vi "Add Authentication.vi"(7 "WSDL URL":string, 8 "error in (no error)":errorcluster, 9 "Proxy Server Settings":T1, 10 "Web Service Authentication":T2, 11 "SoapHttpClientProtocolIn":refnum<k24>) -> (0 "error out":errorcluster, 3 "SoapHttpClientProtocolOut":refnum<k24>)   [LabVIEW 2017, in "WebServiceImporter.lvlib" / "VI Generator.lvlib"]
uses:
  <vilib>/Platform/WebService/VI Generator/VI Generator.lvlib
  System.Web.Services
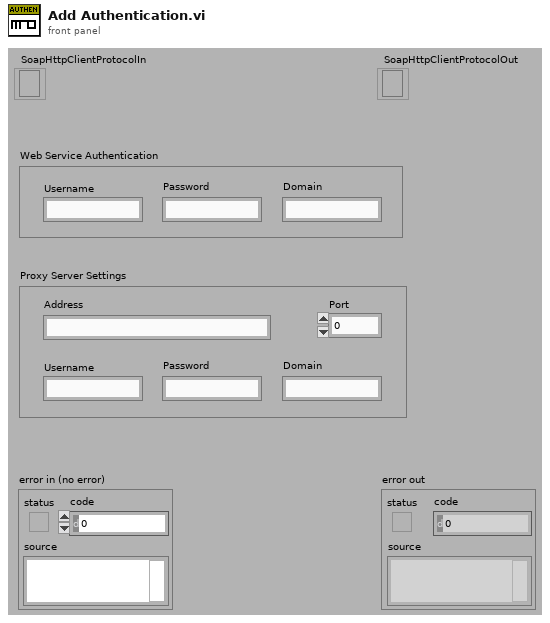
[diagram p1: front panel]
types:
  T1 = cluster{"Address":string, "Port":u32, "Username":string, "Password":string, "Domain":string}
  T2 = cluster{"Username":string, "Password":string, "Domain":string}
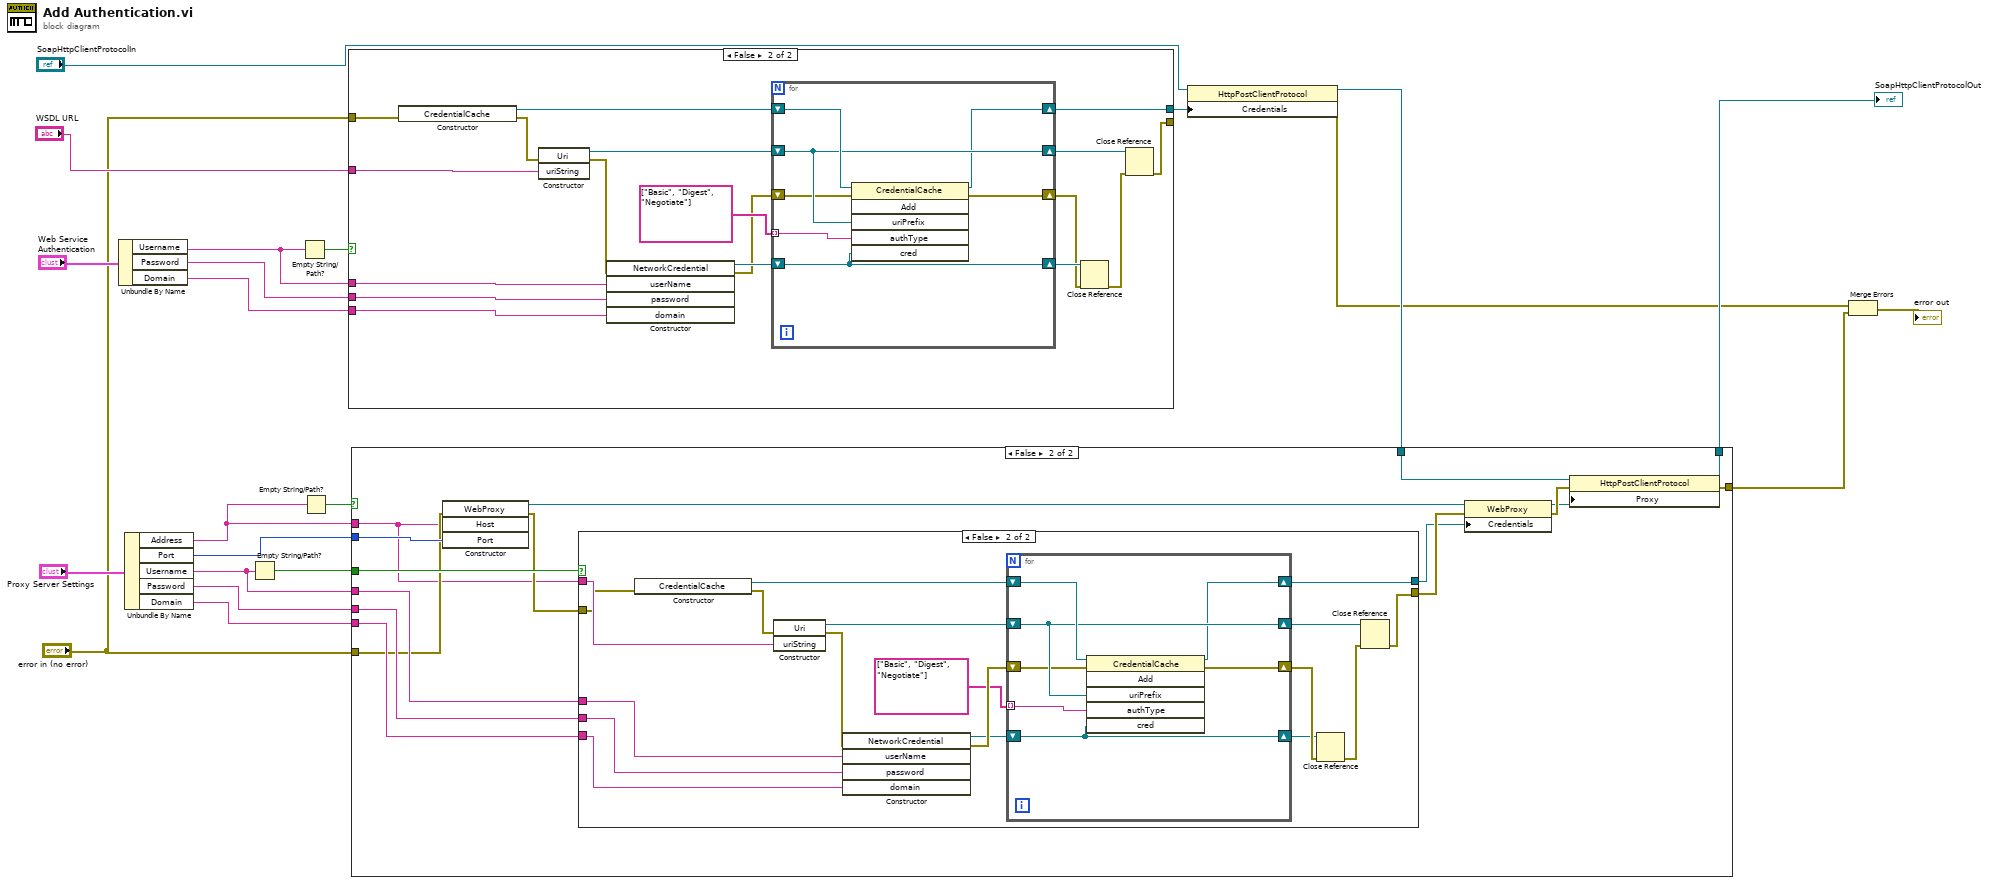
[diagram p0: block diagram]
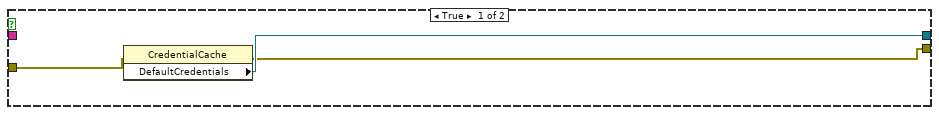
[diagram p3: hidden frame]
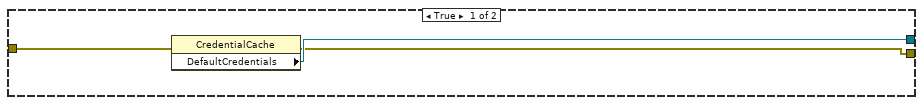
[diagram p4: hidden frame]
diagram:
  n1 = Unbundle By Name("Web Service Authentication") -> ("Username"=w18:string, "Password"=w17:string, "Domain"=w16:string)
  n2 = Unbundle By Name("Proxy Server Settings") -> ("Address"=w12:string, "Port"=w11:u32, "Username"=w7:string, "Password"=w9:string, "Domain"=w8:string)
  n3 = Empty String/Path?(string/path=w7) -> (empty?=w10:bool)
  n4 = Empty String/Path?(string/path=w18) -> (empty?=w20:bool)
  n5 = Empty String/Path?(string/path=w12) -> (empty?=w13:bool)
  n6 = case shown="False" w20 {
    tunnel: "error in (no error)" -> [w25 w43]
    tunnel: "WSDL URL" -> [_ w41]
    tunnel: w18 -> [_ w40]
    tunnel: w17 -> [_ w39]
    tunnel: w16 -> [_ w38]
    tunnel: [w23 w27] -> _
    tunnel: [w24 w26] -> w14
    frame True {
      n7 = property class="CredentialCache"(error in=w25) -> (error out=w23:errorcluster, "DefaultCredentials"=w24:refnum<k24>)  [unwired: 1 in, 1 out]
    }
    frame False {
      n8 = constructor class="CredentialCache"(error in=w43) -> (reference out=w35:refnum<k24>, error out=w42:errorcluster)  [unwired: 2 in, 1 out]
      n9 = constructor class="Uri"(error in=w42, "uriString"=w41) -> (reference out=w34:refnum<k24>, error out=w37:errorcluster)  [unwired: 2 in, 2 out]
      n10 = constructor class="NetworkCredential"(error in=w37, "userName"=w40, "password"=w39, "domain"=w38) -> (reference out=w33:refnum<k24>, error out=w32:errorcluster)  [unwired: 2 in, 4 out]
      n11 = for {
        tunnel: string[] ["Basic", "Digest", "Negotiate"] -> [w45] mode=indexing
        shift-right: [w46] -> w28
        shift-left: w32 -> [w47]
        shift-right: [w49] -> w30
        shift-left: w34 -> [w49]
        shift-right: [w48] -> w26
        shift-left: w35 -> [w50]
        shift-right: [w44] -> w31
        shift-left: w33 -> [w44]
        n12 = invoke class="CredentialCache" method="Add"(reference=w50, error in=w47, "uriPrefix"=w49, "authType"=w45, "cred"=w44) -> (reference out=w48:refnum<k24>, error out=w46:errorcluster)  [unwired: 1 in, 4 out]
      }
      n13 = Close Reference(reference=w31, error in (no error)=w28) -> (error out=w29:errorcluster)
      n14 = Close Reference(reference=w30, error in (no error)=w29) -> (error out=w27:errorcluster)
    }
  }
  n15 = property class="HttpPostClientProtocol"(reference="SoapHttpClientProtocolIn", "Credentials"=w14) -> (reference out=w5:refnum<k24>, error out=w3:errorcluster)  [unwired: 1 in]
  n16 = case shown="False" w13 {
    tunnel: w12 -> [_ w61]
    tunnel: w11 -> [_ w68]
    tunnel: w10 -> [_ w67]
    tunnel: w9 -> [_ w65]
    tunnel: w8 -> [_ w64]
    tunnel: w7 -> [_ w66]
    tunnel: "error in (no error)" -> [w51 w63]
    tunnel: w5 -> [w52 w57]
    tunnel: [w52 w55] -> w4
    tunnel: [w51 w54] -> w2
    frame True {
    }
    frame False {
      n17 = constructor class="WebProxy"(error in=w63, "Host"=w61, "Port"=w68) -> (reference out=w58:refnum<k24>, error out=w62:errorcluster)  [unwired: 2 in, 3 out]
      n18 = case shown="False" w67 {
        tunnel: w66 -> [_ w76]
        tunnel: w65 -> [_ w75]
        tunnel: w64 -> [_ w74]
        tunnel: w62 -> [w71 w77]
        tunnel: w61 -> [_ w78]
        tunnel: [w69 w73] -> w60
        tunnel: [w70 w72] -> w59
        frame True {
          n19 = property class="CredentialCache"(error in=w71) -> (error out=w69:errorcluster, "DefaultCredentials"=w70:refnum<k24>)  [unwired: 1 in, 1 out]
        }
        frame False {
          n20 = constructor class="CredentialCache"(error in=w77) -> (reference out=w82:refnum<k24>, error out=w79:errorcluster)  [unwired: 2 in, 1 out]
          n21 = constructor class="Uri"(error in=w79, "uriString"=w78) -> (reference out=w83:refnum<k24>, error out=w80:errorcluster)  [unwired: 2 in, 2 out]
          n22 = constructor class="NetworkCredential"(error in=w80, "userName"=w76, "password"=w75, "domain"=w74) -> (reference out=w84:refnum<k24>, error out=w85:errorcluster)  [unwired: 2 in, 4 out]
          n23 = for {
            tunnel: string[] ["Basic", "Digest", "Negotiate"] -> [w91] mode=indexing
            shift-right: [w92] -> w89
            shift-left: w85 -> [w93]
            shift-right: [w95] -> w87
            shift-left: w83 -> [w95]
            shift-right: [w94] -> w72
            shift-left: w82 -> [w96]
            shift-right: [w90] -> w86
            shift-left: w84 -> [w90]
            n24 = invoke class="CredentialCache" method="Add"(reference=w96, error in=w93, "uriPrefix"=w95, "authType"=w91, "cred"=w90) -> (reference out=w94:refnum<k24>, error out=w92:errorcluster)  [unwired: 1 in, 4 out]
          }
          n25 = Close Reference(reference=w86, error in (no error)=w89) -> (error out=w88:errorcluster)
          n26 = Close Reference(reference=w87, error in (no error)=w88) -> (error out=w73:errorcluster)
        }
      }
      n27 = property class="WebProxy"(reference=w58, error in=w60, "Credentials"=w59) -> (reference out=w53:refnum<k24>, error out=w56:errorcluster)
      n28 = property class="HttpPostClientProtocol"(reference=w57, error in=w56, "Proxy"=w53) -> (reference out=w55:refnum<k24>, error out=w54:errorcluster)
    }
  }
  "SoapHttpClientProtocolOut" <- w4
  n29 = Merge Errors(w3, w2) -> (→"error out":errorcluster)
